vi "Left Variables.vi"() -> ()   [LabVIEW 2015]
panel:
  in  "L o2 X Center":u16
  in  "L o2 Y Center":u16
  in  "L o1 X Center":u16
  in  "L o1 Y Center":u16
  in  "LB Tracked?":bool
  in  "L Avg TB X Center":dbl
  in  "L Avg TB Y Center":dbl
  in  "L Raw TB X Center":u16
  in  "L Raw TB Y Center":u16
  in  "L Left Beacon Angle":dbl
  in  "L Right Beacon Angle":dbl
  in  "L Tilt Pulse Width":u32
  in  "L Run Tilt Motor":bool
  in  "L Unknown Beacon Angle 1":dbl
  in  "L Unknown Beacon Angle 2":dbl
  in  "L Data Valid?":bool
  in  "L Pan Pulse Width":u32
  in  "Heading":dbl
  in  "Center X":dbl
  in  "Center Y":dbl
  in  "rcx":dbl
  in  "rcy":dbl
  in  "lcx":dbl
  in  "lcy":dbl
  in  "L Run Pan Motor":bool
  in  "Beacon Radius":dbl
  in  "Robot Length (rs)":dbl
  in  "Trough Length (ts)":dbl
  in  "L Y Avg":bool
  in  "L X Avg":bool
  in  "L Avg RB X Center":dbl
  in  "L Avg RB Y Center":dbl
  in  "L Avg LB X Center":dbl
  in  "L Avg LB Y Center":dbl
  in  "L STOP":bool
  in  "L Avg Distance (ft)":dbl
  in  "LT Stable":bool
  in  "LP Stable":bool
  in  "LT Limit Reached":bool
  in  "L State":string
  in  "L Avg Zone":dbl
  in  "L Raw RB X Center":u16
  in  "L Raw RB Y Center":u16
  in  "L Raw LB X Center":u16
  in  "L Raw LB Y Center":u16
  in  "LP Limit Reached":bool
  in  "L Dec Speed Zone":dbl
  in  "L Pan Angle":dbl
  in  "L Tilt Angle":dbl
  in  "L Pan Direction":bool
  in  "L Tilt Direction":bool
  in  "L Distance (in)":dbl
  in  "L Distance (ft)":dbl
  in  "L Distance (cm)":dbl
  in  "L Tilt Upper Limit":u16
  in  "L Tilt Lower Limit":u16
  in  "L Pan Upper Limit":u16
  in  "L Pan Lower Limit":u16
  in  "L Default Pulse Width":u32
  in  "L Pan Count":i32
  in  "L Tilt Count":i32
  # "Calculated\nCorner\nCoordinates"
  # "Final\nLocalization\nData"
  # "RAW + AVG\nLIDAR\nData"
  # "o1\no2\n( X , Y )"
  # "AVG\nBeacon\n( X , Y )"
  # "TRACKED\nBeacon\n( X , Y )"
  # "RAW\nBeacon\n( X , Y )"
  # "Motor\nStep\nCounts"
  # "Motor\nPosition\nAngles"
  # "Unknown\nBeacon\nAngles"
  # "Deduced\nBeacon\nAngles"
  # "Known\nConstants"
  # "Tracking\nDead Zone\nLimits"
  # "Special\nTracking Zone\nDomains"
  # "Motor\nPulse\nWidths"
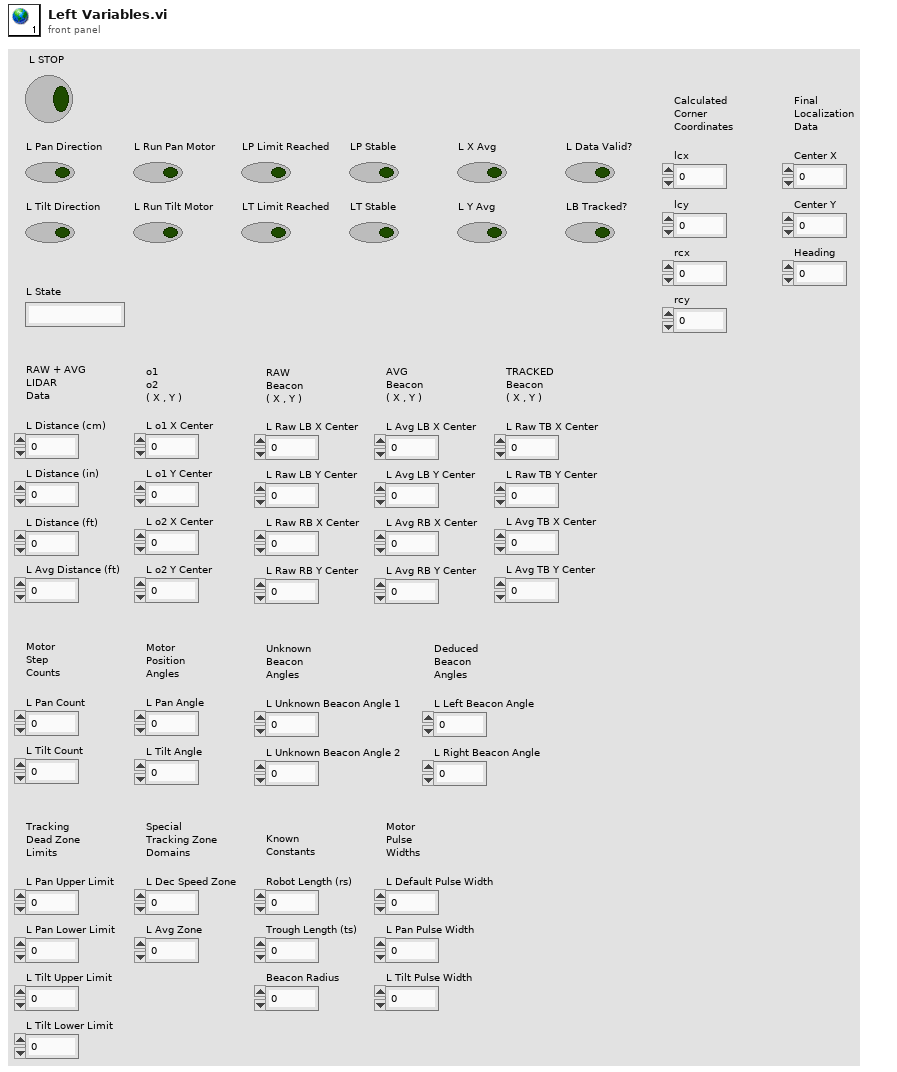
[diagram p1: front panel]
diagram:
